vi "CHANNEL VALUES.vi"(6 "Channel no":dbl, 8 "VISA resource":refnum<visa-resource-name>="COM5", 9 "Enum":enum16{"CHANNEL", "INDEX"}(ring)) -> (1 "Channel Out":u32)   [LabVIEW 2021]
uses:
  <vilib>/Instr/_visa.llb/VISA Configure Serial Port (Instr).vi
panel:
  out "output array":u8[](array[numeric])
  out "error out":errorcluster
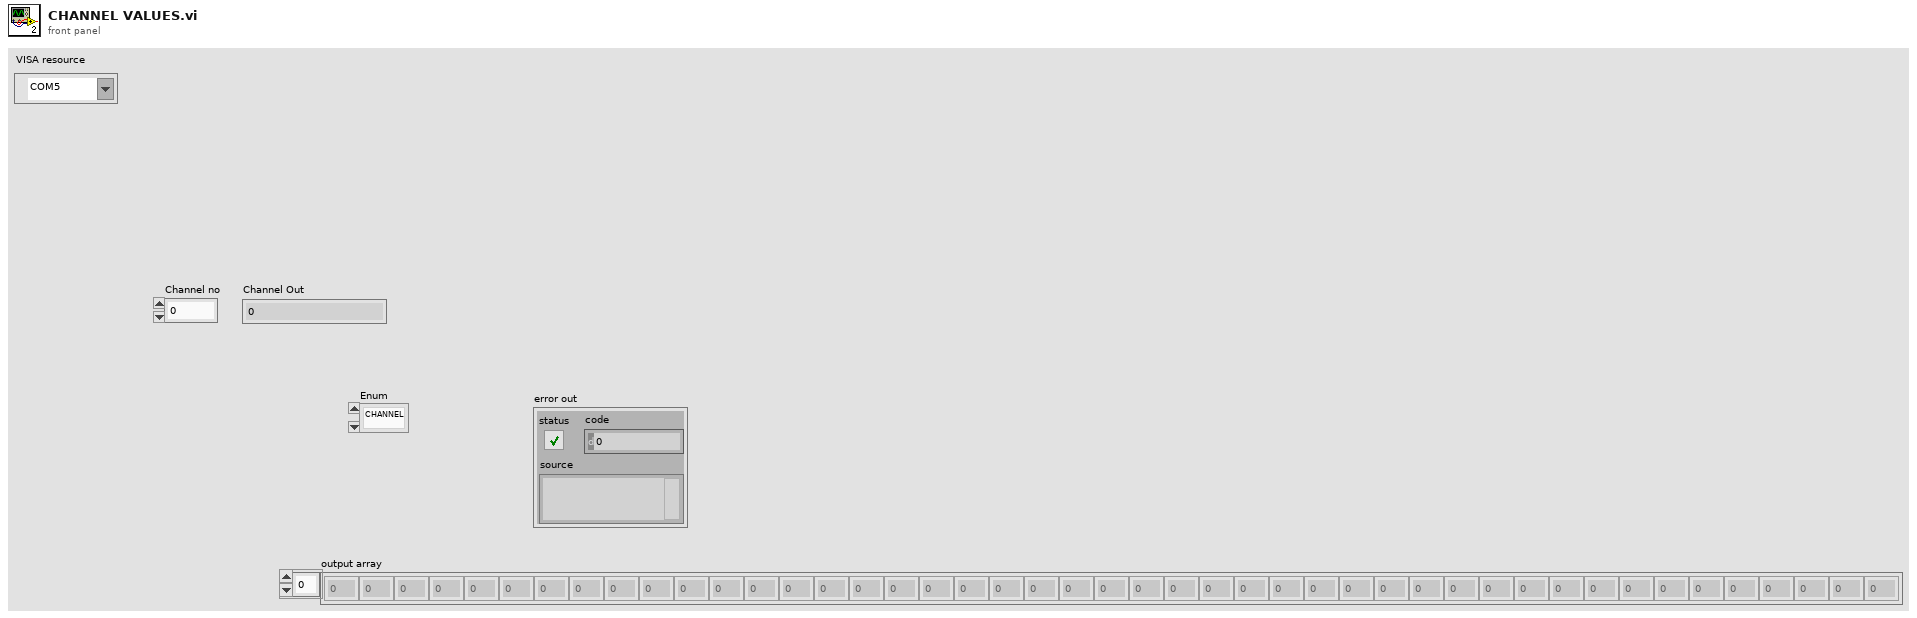
[diagram p1: front panel]
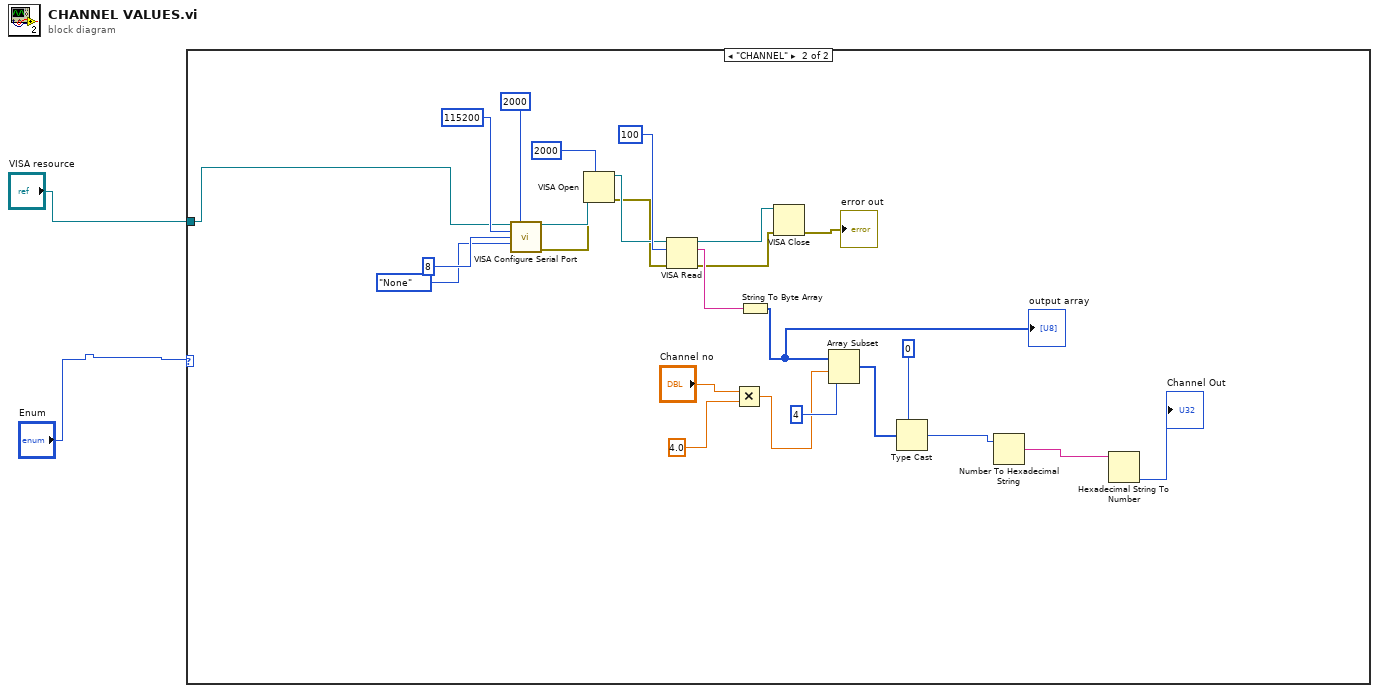
[diagram p0: block diagram]
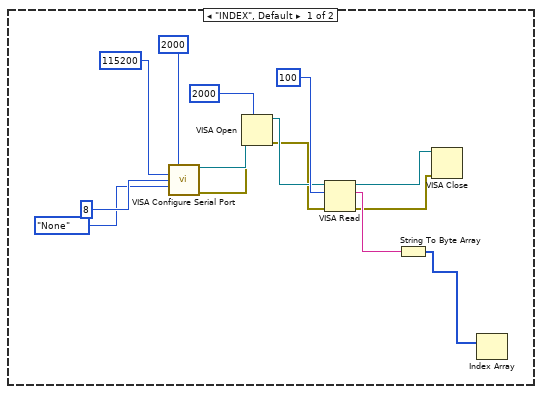
[diagram p2: hidden frame]
diagram:
  n1 = case shown="\"CHANNEL\"" "Enum" {
    tunnel: "VISA resource" -> [_ w17]
    frame "INDEX", Default {
      n2 = call-poly "VISA Configure Serial Port"("timeout (10sec)"=u32 2000, "baud rate (9600)"=u32 115200, "data bits (8)"=u16 8, "parity (0:none)"=enum16{"None", "Odd", "Even", "Mark", "Space"}."None") -> ("VISA resource name out"=w13:refnum<visa-resource-name>, "error out"=w12:errorcluster)  [unwired: 10 in]
      n3 = VISA Open(timeout (0)=u32 2000 ("VISA Open timeout (0)"), error in (no error)=w12, VISA resource name=w13) -> (VISA resource name=w8:refnum<visa-resource-name>, error out=w7:errorcluster)  [unwired: 2 in]
      n4 = VISA Read(VISA resource name=w8, byte count=u32 100, error in (no error)=w7) -> (VISA resource name out=w5:refnum<visa-resource-name>, read buffer=w6:string, error out=w4:errorcluster)  [unwired: 1 out]
      n5 = String To Byte Array(string=w6) -> (unsigned byte array=w3:u8[])
      n6 = VISA Close(VISA resource name=w5, error in (no error)=w4) -> ()  [unwired: 1 out]
      n7 = Index Array(array=w3) -> ()  [unwired: 1 in, 1 out]
    }
    frame "CHANNEL" {
      n8 = call-poly "VISA Configure Serial Port"("VISA resource name"=w17, "timeout (10sec)"=u32 2000, "baud rate (9600)"=u32 115200, "data bits (8)"=u16 8, "parity (0:none)"=enum16{"None", "Odd", "Even", "Mark", "Space"}."None") -> ("VISA resource name out"=w37:refnum<visa-resource-name>, "error out"=w36:errorcluster)  [unwired: 9 in]
      n9 = VISA Open(timeout (0)=u32 2000 ("VISA Open timeout (0)"), error in (no error)=w36, VISA resource name=w37) -> (VISA resource name=w32:refnum<visa-resource-name>, error out=w31:errorcluster)  [unwired: 2 in]
      n10 = VISA Read(VISA resource name=w32, byte count=u32 100, error in (no error)=w31) -> (VISA resource name out=w19:refnum<visa-resource-name>, read buffer=w21:string, error out=w18:errorcluster)  [unwired: 1 out]
      n11 = Multiply(x="Channel no", y=4.0) -> (x*y=w25:dbl)
      n12 = String To Byte Array(string=w21) -> (unsigned byte array=w20:u8[])
      "output array" <- w20
      n13 = VISA Close(VISA resource name=w19, error in (no error)=w18) -> (error out=→"error out":errorcluster)
      n14 = Array Subset(array=w20, index=w25, length=4) -> (w22:u8[])
      n15 = Type Cast(type=0, x=w22) -> (*(type *) &x=w28:i32)
      n16 = Number To Hexadecimal String(2:w28) -> (0:w24:string)  [unwired: 1 in]
      n17 = Hexadecimal String To Number(string=w24) -> (number=→"Channel Out":u32)  [unwired: 2 in, 1 out]
    }
  }
